vi "SVM_op_range_exp.vi"() -> ()   [LabVIEW 2013]
doc: "This VI runs the experiment that is used to build the operating range SVM for the burner system."
uses:
  Controls/pressure_control_cluster.ctl
  Controls/run_mode_enum.ctl
  Controls/Fitz9_pressure_indicator_cluster.ctl
panel:
  in  "Flame":bool
  out "Pressure Indicators":T1
  in  "Pressure Controls":T2={"Atm Press"=0.0, "Des P drop"=0.0, "Phi"=0.0, "PID gains"={"proportional gain (Kc)"=3.0, "integral time (Ti, min)"=0.0003, "derivative time (Td, min)"=-0.0001}, "output range"={"output high"=400.0, "output low"=0.0}, "Run Mode"=enum."Non pre-mixed"} {"output range"."output low" format="%.2f"; "output range"."output high" format="%.2f"; "PID gains"."derivative time (Td, min)" format="%.6f"; "PID gains"."integral time (Ti, min)" format="%.5f"; "PID gains"."proportional gain (Kc)" format="%.3f"; "Phi" scale=0.0..1.5; "Des P drop" scale=0.0..6.0}
  out "Arg. Array":dbl[](array[numeric])
  out "Output path":string caption="Output File Name"
  out "Flame?":bool
  out "Test path":string caption="Test Specification Name"
  in  "Run Exp.":bool
  in  "Open File":bool
  in  "Stop Button":bool
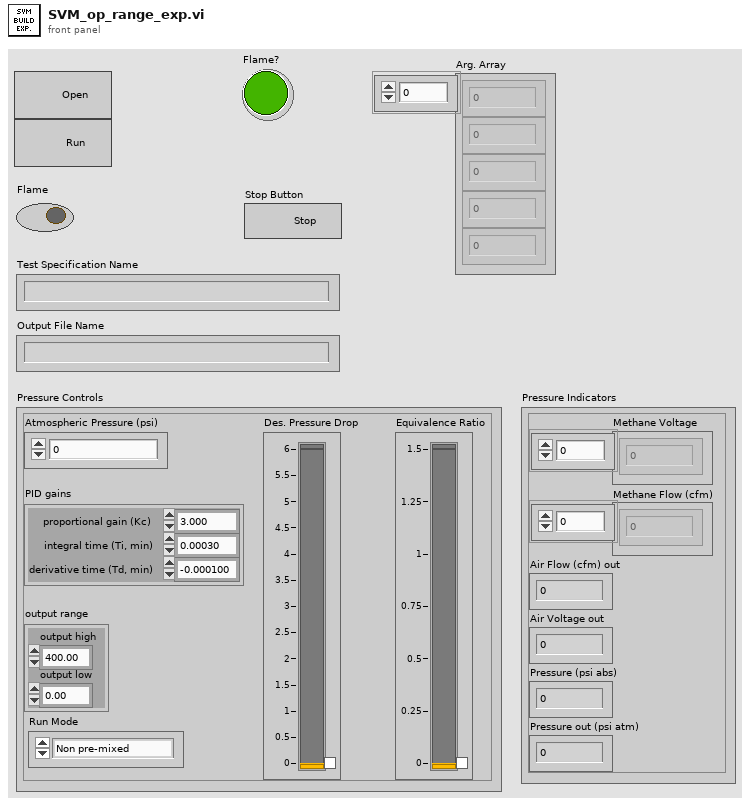
[diagram p1: front panel]
types:
  T1 = typedef "Fitz9_pressure_indicator_cluster.ctl" = cluster{"Methane Voltage":dbl[], "Methane Flow (cfm)":dbl[], "Air Flow (cfm) out":dbl, "Air Voltage out":dbl, "Pressure (psi abs)":dbl, "Pressure out (psi atm)":dbl}
  T2 = typedef "pressure_control_cluster.ctl" = cluster{"Atm Press":dbl, "Des P drop":dbl, "Phi":dbl, "PID gains":cluster{"proportional gain (Kc)":dbl, "integral time (Ti, min)":dbl, "derivative time (Td, min)":dbl}, "output range":cluster{"output high":dbl, "output low":dbl}, "Run Mode":T3}
  T3 = typedef "run_mode_enum.ctl" = enum16{"Non pre-mixed", "Pre-mixed"}
  T4 = enum16{"open", "replace", "create", "open or create", "replace or create", "replace or create with confirmation"}
  T5 = typedef "timer_input_cluster.ctl" = cluster{"Target Time":dbl, "relight?":bool, "flame?":bool}
  T6 = typedef "timer_output_cluster.ctl" = cluster{"target reached?":bool, "flame out?":bool, "flame lit?":bool}
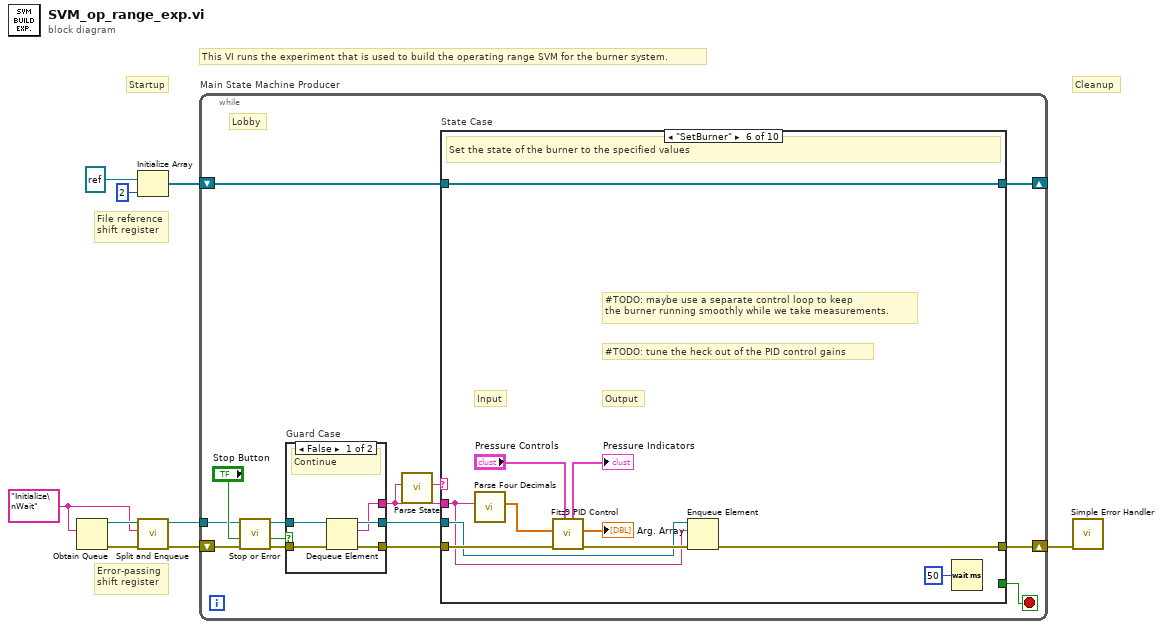
[diagram p0: block diagram]
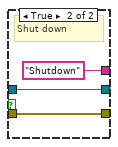
[diagram p2: hidden frame]
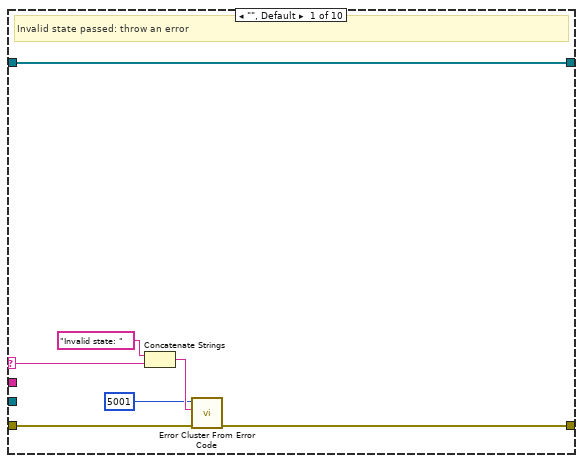
[diagram p3: hidden frame]
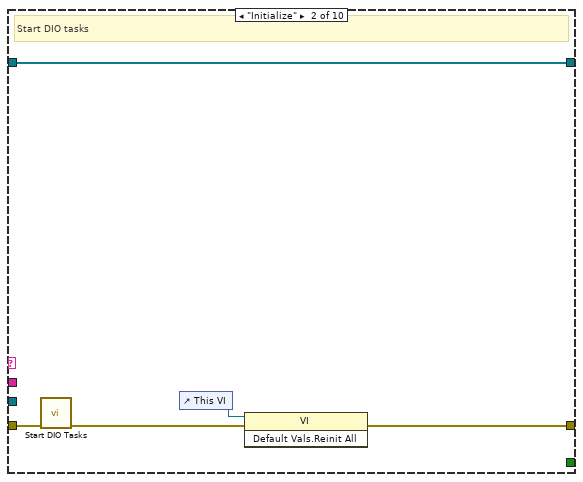
[diagram p4: hidden frame]
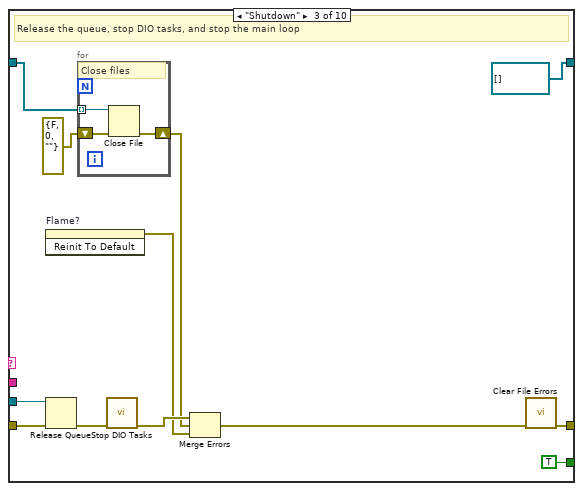
[diagram p5: hidden frame]
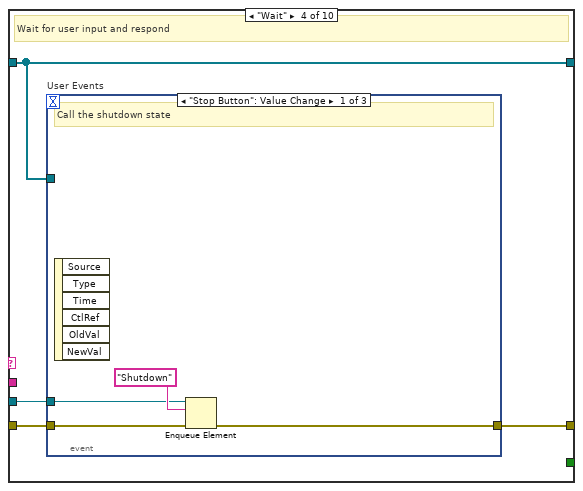
[diagram p6: hidden frame]
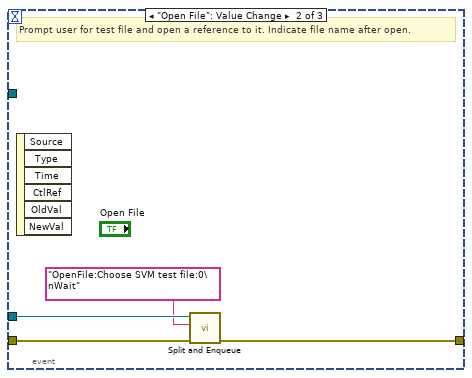
[diagram p7: hidden frame]
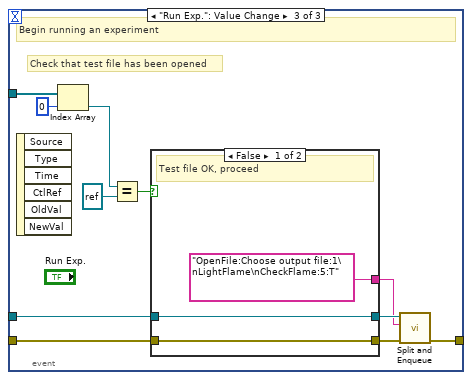
[diagram p8: hidden frame]
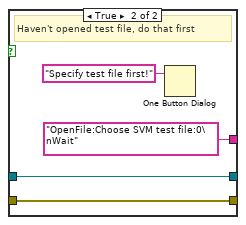
[diagram p9: hidden frame]
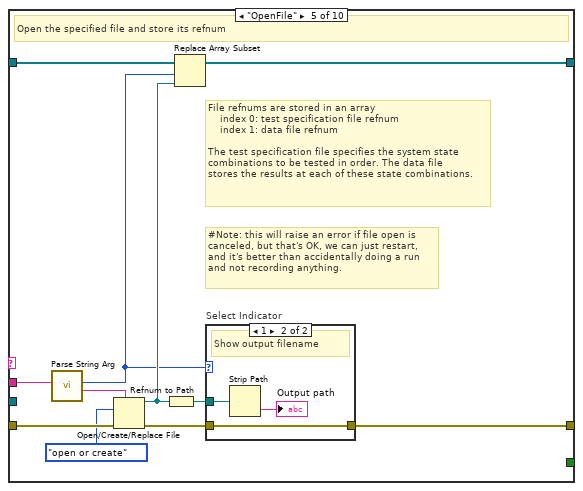
[diagram p10: hidden frame]
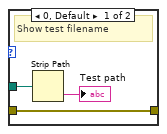
[diagram p11: hidden frame]
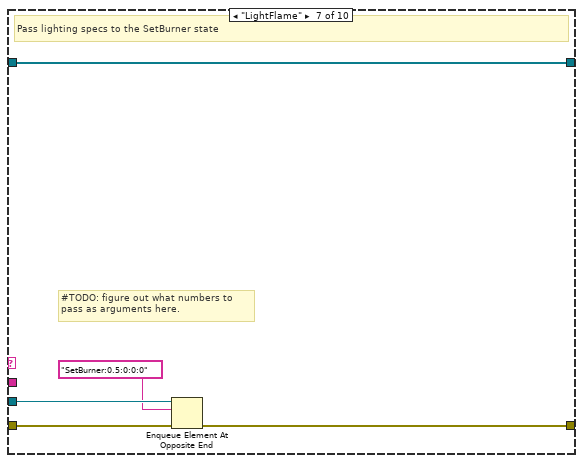
[diagram p12: hidden frame]
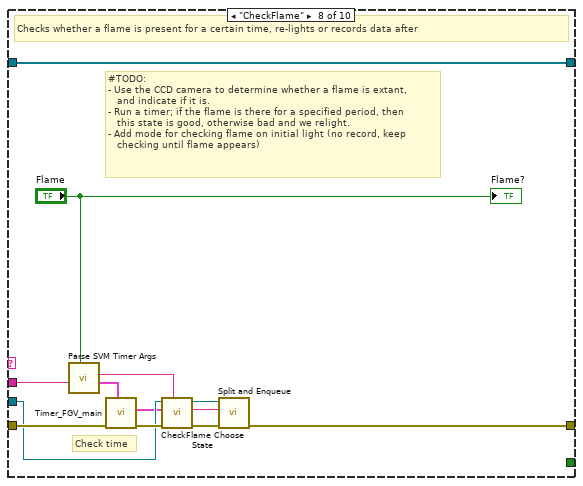
[diagram p13: hidden frame]
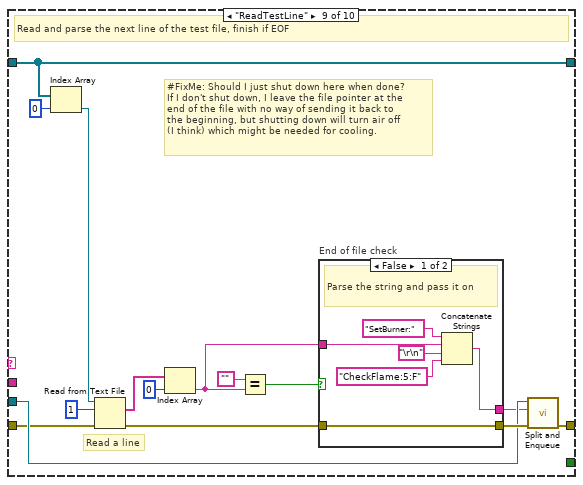
[diagram p14: hidden frame]
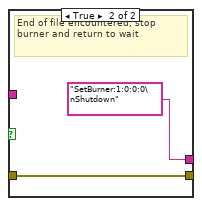
[diagram p15: hidden frame]
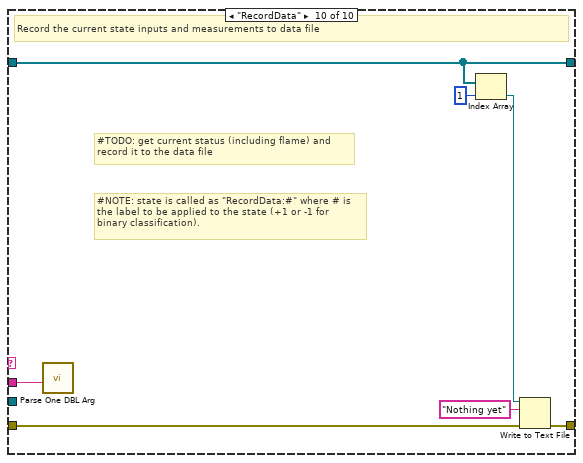
[diagram p16: hidden frame]
diagram:
  w4 = "Initialize\nWait"
  # "File reference\nshift register"
  # "Cleanup"
  # "Startup"
  # "Error-passing\nshift register"
  # "This VI runs the experiment that is used to build the operating range SVM for the burner system."
  n1 = Obtain Queue(element data type=w4) -> (queue out=w7:refnum<queue>, error out=w9:errorcluster)  [unwired: 4 in, 1 out]
  n2 = Initialize Array(refnum<file> refnum ("refnum out"), 2 ("dimension size")) -> (w1:refnum<file>[])
  n3 = call "Split and Enqueue.vi"("error in (no error)"=w9, "Input String"=w4, "queue in"=w7) -> ("error out"=w8:errorcluster, "queue out"=w6:refnum<queue>)  [unwired: 7 in]
  n4 = while "Main State Machine Producer" {
    shift-right: [w17] -> w5
    shift-left: w8 -> [w20]
    tunnel: w6 -> [w16]
    shift-right: [w12] -> _
    shift-left: w1 -> [w11]
    stop <- w13 stop-if-true
    # "Lobby"
    n5 = call "Stop or Error.vi"("Error In"=w20, "Stop Button"="Stop Button") -> ("Error Out"=w19:errorcluster, "Stop or Error?"=w21:bool)  [unwired: 8 in]
    n6 = case "Guard Case" shown="False" w21 {
      tunnel: w19 -> [w27 w29]
      tunnel: [w26 w29] -> w18
      tunnel: w16 -> [w25 w30]
      tunnel: [w24 w30] -> w15
      tunnel: [w23 "Shutdown"] -> w10
      frame False {
        # "Continue"
        n7 = Dequeue Element(queue=w25, error in (no error)=w27) -> (queue out=w24:refnum<queue>, element=w23:string, error out=w26:errorcluster)  [unwired: 1 in, 1 out]
      }
      frame True {
        # "Shut down"
      }
    }
    n8 = call "Parse State.vi"("String with Args"=w10) -> ("State"=w14:string)  [unwired: 10 in]
    n9 = case "State Case" shown="\"SetBurner\"" w14 {
      selector: w14 -> [w34 _ _ _ _ _ _ _ _ _]
      tunnel: w18 -> [w37 w42 w54 w61 w97 w114 w119 w129 w135 w162]
      tunnel: [w36 w38 w43 w60 w95 w108 w118 w131 w142 w163] -> w17
      tunnel: w15 -> [_ _ w52 w59 _ w107 w117 w123 w141 _]
      tunnel: [_ _ TRUE _ _ _ _ _ _ _] -> w13
      tunnel: w10 -> [_ _ _ _ w96 w106 _ w125 _ w157]
      tunnel: [w31 w41 refnum<file>[] [] w58 w92 w115 w120 w133 w148 w161] -> w12
      tunnel: w11 -> [w31 w41 w49 w58 w94 w115 w120 w133 w148 w161]
      frame "", Default {
        # "Invalid state passed: throw an error"
        n10 = Concatenate Strings("Invalid state: " ("string"), w34) -> (w33:string)
        n11 = call <vilib>:"Error Cluster From Error Code.vi"("error in (no error)"=w37, "error message (\"\")"=w33, "error code (0)"=5001) -> ("error out"=w36:errorcluster)  [unwired: 6 in]
      }
      frame "Initialize" {
        # "Start DIO tasks"
        n12 = call "Start DIO Tasks.vi"("error in (no error)"=w42) -> ("error out"=w39:errorcluster)  [unwired: 10 in]
        n13 = control-ref of="This VI"() -> (w40:refnum<vi>)
        n14 = invoke class="VI" method="Default Vals.Reinit All"(reference=w40, error in=w39) -> (error out=w38:errorcluster)  [unwired: 1 in, 2 out]
      }
      frame "Shutdown" {
        # "Release the queue, stop DIO tasks, and stop the main loop"
        n15 = invoke on="Flame?" class="Bool (strict)" method="Reinit To Default"() -> (error out=w45:errorcluster)  [unwired: 3 in, 2 out]
        n16 = Release Queue(queue=w52, error in (no error)=w54) -> (error out=w53:errorcluster)  [unwired: 1 in, 2 out]
        n17 = for {
          tunnel: w49 -> [w57] mode=indexing
          shift-right: [w56] -> w47
          shift-left: errorcluster {"status"=FALSE, "code"=0, "source"=""} ("error constant") -> [w55]
          # "Close files"
          n18 = Close File(refnum=w57, error in=w55) -> (error out=w56:errorcluster)  [unwired: 1 out]
        }
        n19 = call "Stop DIO Tasks.vi"("Error In"=w53) -> ("error out"=w48:errorcluster)  [unwired: 10 in]
        n20 = Merge Errors(w48, w47, w45) -> (w44:errorcluster)
        n21 = call "Clear File Errors.vi"("Error In"=w44) -> ("Error Out"=w43:errorcluster)  [unwired: 10 in]
      }
      frame "Wait" {
        # "Wait for user input and respond"
        n22 = event "User Events" shown="[0] \"Stop Button\": Value Change" {
          selector: _ -> [_ _ _]
          dyn-events: _ -> [_ _ _]
          timeout: _ -> [_ _ _]
          tunnel: w61 -> [w65 w69 w75]
          tunnel: [w64 w67 w73] -> w60
          tunnel: w59 -> [w62 w68 w74]
          tunnel: w58 -> [_ _ w80]
          event "Stop Button": Value Change {
            # "Call the shutdown state"
            n23 = event-data() -> ()  [unwired: 1 in, 6 out]
            n24 = Enqueue Element(queue=w62, element="Shutdown", error in (no error)=w65) -> (error out=w64:errorcluster)  [unwired: 1 in, 2 out]
          }
          event "Open File": Value Change {
            # "Prompt user for test file and open a reference to it. Indicate file name after open."
            n25 = event-data() -> ()  [unwired: 1 in, 6 out]
            n26 = call "Split and Enqueue.vi"("error in (no error)"=w69, "Input String"="OpenFile:Choose SVM test file:0\nWait", "queue in"=w68) -> ("error out"=w67:errorcluster)  [unwired: 7 in, 1 out]
          }
          event "Run Exp.": Value Change {
            # "Check that test file has been opened"
            # "Begin running an experiment"
            n27 = event-data() -> ()  [unwired: 1 in, 6 out]
            n28 = Index Array(array=w80, index=0) -> (element=w78:refnum<file>)
            n29 = Equal?(x=w78, y=refnum<file> refnum ("refnum out")) -> (x = y?=w76:bool)
            n30 = case shown="False" w76 {
              tunnel: w75 -> [w81 w87]
              tunnel: w74 -> [w82 w86]
              tunnel: [w81 w87] -> w72
              tunnel: [w82 w86] -> w71
              tunnel: ["OpenFile:Choose output file:1\nLightFlame\nCheckFlame:5:T" ("Input String") "OpenFile:Choose SVM test file:0\nWait" ("Input String")] -> w70
              frame False {
                # "Test file OK, proceed"
              }
              frame True {
                # "Haven't opened test file, do that first"
                n31 = One Button Dialog(message="Specify test file first!") -> ()  [unwired: 1 in, 1 out]
              }
            }
            n32 = call "Split and Enqueue.vi"("error in (no error)"=w72, "Input String"=w70, "queue in"=w71) -> ("error out"=w73:errorcluster)  [unwired: 7 in, 1 out]
          }
        }
      }
      frame "OpenFile" {
        # "#Note: this will raise an error if file open is\ncanceled, but that's OK, we can just restart,\nand it's better than accidentally doing a run\nand not recording anything."
        # "File refnums are stored in an array\n    index 0: test specification file refnum\n    index 1: data file refnum\n\nThe test specification file specifies the system state\ncombinations to be tested in order. The data file\nstores the results at each of these state combinations."
        # "Open the specified file and store its refnum"
        n33 = call "Parse String Arg.vi"("Input String"=w96) -> ("String Arg"=w89:string, "Integer Out"=w88:i32)  [unwired: 9 in]
        n34 = Open/Create/Replace File(error in=w97, prompt=w89, operation (0:open)=T4."open or create") -> (refnum out=w93:refnum<file>, error out=w98:errorcluster)  [unwired: 3 in, 1 out]
        n35 = Refnum to Path(1:w93) -> (0:w90:path)
        n36 = Replace Array Subset(array=w94, new element=w93, index=w88) -> (w92:refnum<file>[])
        n37 = case "Select Indicator" shown="1" w88 {
          tunnel: w90 -> [w100 w103]
          tunnel: w98 -> [w101 w104]
          tunnel: [w101 w104] -> w95
          frame 0, Default {
            # "Show test filename"
            n38 = Strip Path(path=w100) -> (name=→"Test path":string)  [unwired: 1 out]
          }
          frame 1 {
            # "Show output filename"
            n39 = Strip Path(path=w103) -> (name=→"Output path":string)  [unwired: 1 out]
          }
        }
      }
      frame "SetBurner" {
        # "Output"
        # "Input"
        # "#TODO: tune the heck out of the PID control gains"
        # "#TODO: maybe use a separate control loop to keep\nthe burner running smoothly while we take measurements."
        # "Set the state of the burner to the specified values"
        n40 = call "Parse Four Decimals.vi"("Input String"=w106) -> ("Arg. Array"=w112:dbl[])  [unwired: 10 in]
        n41 = call "Fitz9 PID Control.vi"("Pressure Controls"="Pressure Controls", "Error In"=w114, "Set Point Array"=w112) -> ("Error Out"=w113:errorcluster, "Set Point Array out"=→"Arg. Array":dbl[], "Pressure Indicators"=→"Pressure Indicators":T1)  [unwired: 6 in]
        n42 = Enqueue Element(queue=w107, element=w106, error in (no error)=w113) -> (error out=w108:errorcluster)  [unwired: 1 in, 2 out]
        n43 = Wait (ms)(milliseconds to wait=u32 50) -> ()  [unwired: 1 out]
      }
      frame "LightFlame" {
        # "#TODO: figure out what numbers to\npass as arguments here."
        # "Pass lighting specs to the SetBurner state"
        n44 = Enqueue Element At Opposite End(queue=w117, element="SetBurner:0.5:0:0:0", error in (no error)=w119) -> (error out=w118:errorcluster)  [unwired: 1 in, 2 out]
      }
      frame "CheckFlame" {
        # "Check time"
        # "#TODO:\n- Use the CCD camera to determine whether a flame is extant,\n   and indicate if it is.\n- Run a timer; if the flame is there for a specified period, then\n   this state is good, otherwise bad and we relight.\n- Add mode for checking flame on initial light (no record, keep\n   checking until flame appears)"
        # "Checks whether a flame is present for a certain time, re-lights or records data after"
        n45 = call "Parse SVM Timer Args.vi"("Flame?"="Flame", "State String"=w125) -> ("Timer Inputs"=w124:T5, "State String out"=w122:string)  [unwired: 8 in]
        n46 = call "Timer_FGV_main.vi"("Timer Inputs"=w124, "Error In"=w129) -> ("Error Out"=w128:errorcluster, "Timer Outputs"=w121:T6)  [unwired: 8 in]
        n47 = call "CheckFlame Choose State.vi"("State String"=w122, "error in"=w128, "Timer Outputs"=w121, "Queue in"=w123) -> ("error out"=w132:errorcluster, "String"=w130:string, "Queue out"=w127:refnum<queue>)  [unwired: 5 in]
        n48 = call "Split and Enqueue.vi"("error in (no error)"=w132, "Input String"=w130, "queue in"=w127) -> ("error out"=w131:errorcluster)  [unwired: 7 in, 1 out]
        "Flame?" <- "Flame"
      }
      frame "ReadTestLine" {
        # "#FixMe: Should I just shut down here when done?\nIf I don't shut down, I leave the file pointer at the\nend of the file with no way of sending it back to\nthe beginning, but shutting down will turn air off\n(I think) which might be needed for cooling."
        # "Read a line"
        # "Read and parse the next line of the test file, finish if EOF"
        n49 = Index Array(array=w148, index=0) -> (element=w139:refnum<file>)
        n50 = Read from Text File(file (use dialog)=w139, count=1, error in=w135) -> (text=w138:string[], error out=w134:errorcluster)  [unwired: 1 in, 2 out]
        n51 = Index Array(array=w138, index=0) -> (element=w136:string)
        n52 = Equal?(x="", y=w136) -> (x = y?=w144:bool)
        n53 = case "End of file check" shown="False" w144 {
          tunnel: [w149 w155] -> w143
          tunnel: w136 -> [w153 _]
          tunnel: [w150 "SetBurner:1:0:0:0\nShutdown"] -> w140
          tunnel: w134 -> [w149 w155]
          frame False {
            # "Parse the string and pass it on"
            n54 = Concatenate Strings("SetBurner:" ("string"), w153, "\r\n", "CheckFlame:5:F" ("string")) -> (w150:string)
          }
          frame True {
            # "End of file encountered, stop burner and return to wait"
          }
        }
        n55 = call "Split and Enqueue.vi"("error in (no error)"=w143, "Input String"=w140, "queue in"=w141) -> ("error out"=w142:errorcluster)  [unwired: 7 in, 1 out]
      }
      frame "RecordData" {
        # "#NOTE: state is called as \"RecordData:#\" where # is\nthe label to be applied to the state (+1 or -1 for\nbinary classification)."
        # "#TODO: get current status (including flame) and\nrecord it to the data file"
        # "Record the current state inputs and measurements to data file"
        n56 = call "Parse One DBL Arg.vi"("State String"=w157) -> ()  [unwired: 10 in, 1 out]
        n57 = Index Array(array=w161, index=1) -> (element=w159:refnum<file>)
        n58 = Write to Text File(file (use dialog)=w159, text="Nothing yet", error in=w162) -> (error out=w163:errorcluster)  [unwired: 1 in, 2 out]
      }
    }
  }
  n59 = call <vilib>:"Simple Error Handler.vi"("error in (no error)"=w5) -> ()  [unwired: 4 in, 5 out]
